vi "HapticSTM3.vi"() -> ()   [LabVIEW 2017]
uses:
  <vilib>/Analysis/baseanly.llb/Mean (DBL).vi
  <userlib>/PositionDLL/PositionDLL.lvlib
  <userlib>/Nanonis Prog Interface V5/Nanonis Prog Interface.lvlib
  <vilib>/Analysis/NI_AALBase.lvlib
panel:
  in  "mean":dbl
  in  "Averaging Done?":bool
  out "Numeric":i32
  out "PLANE HEIGHT":dbl
  out "Current":dbl
  out "Input Z":dbl
  out "Origin Y":dbl
  out "Origin X":dbl
  out "Output Z":dbl
  in  "Rough adjust":dbl
  out "Nano Z":dbl
  out "Y Out":dbl
  out "X Out":dbl
  out "Max speed":dbl
  out "Width":dbl
  out "VY":dbl
  out "VZ":dbl
  out "VX":dbl
  in  "Drag":dbl=1.0
  in  "STOP":bool
  in  "START":bool
  out "Fy":dbl
  out "Fz":dbl
  out "phi":dbl
  out "psi":dbl
  out "Fx":dbl
  out "theta":dbl
  out "x":dbl
  out "y":dbl
  out "z":dbl
  in  "Fine adjust":dbl=3.5
  out "Clicks":dbl
  out "Height":dbl
  # "Sample Window"
  # "Position"
  # "Sensitivity"
  # "Force"
  # "STM I/O"
  # "Angles"
  # "Velocity"
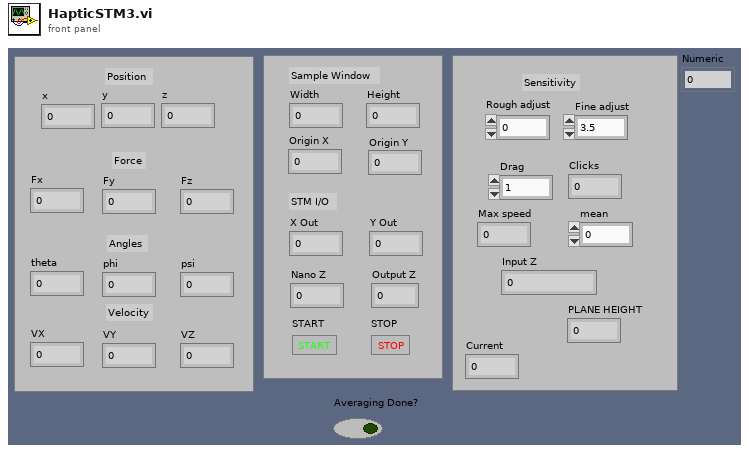
[diagram p1: front panel]
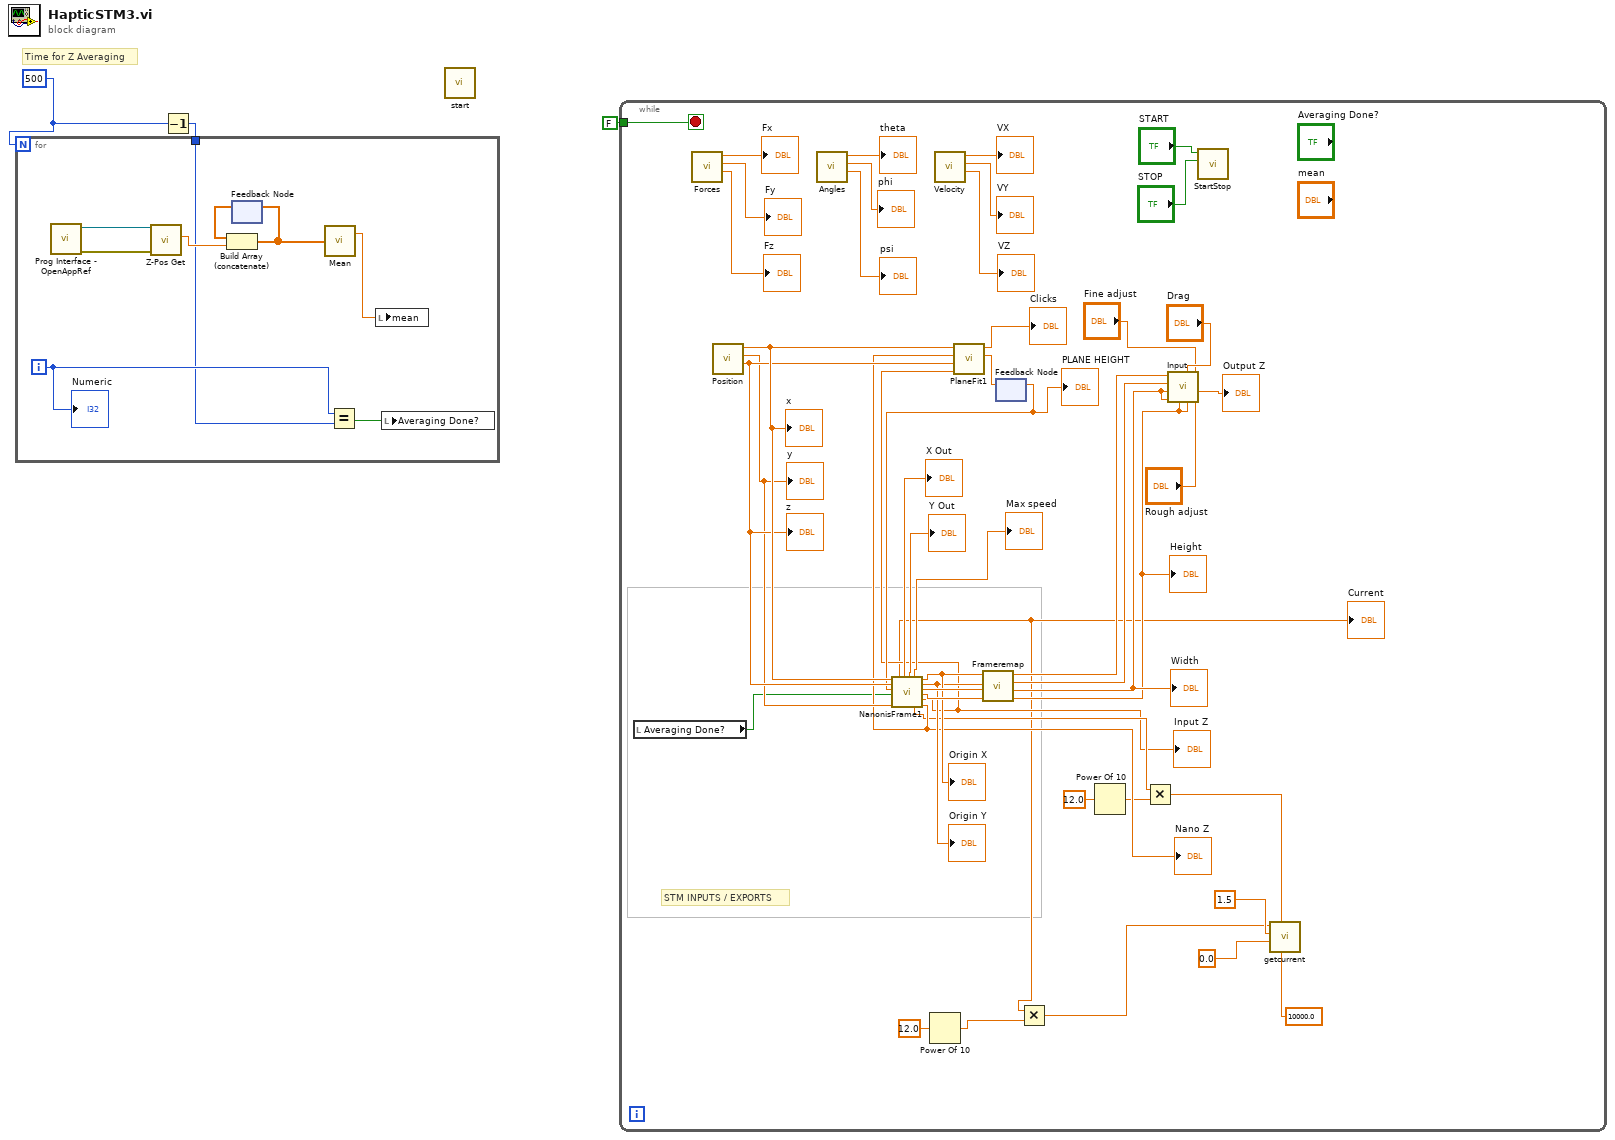
[diagram p0: block diagram]
diagram:
  w2 = 500
  # "Time for Z Averaging"
  n1 = Decrement(x=w2) -> (x-1=w1:i32)
  n2 = for {
    N: w2 -> [_]
    tunnel: w1 -> [w5]
    i -> [w7]
    n3 = call <userlib>:"Prog Interface - OpenAppRef.vi"() -> ("Error out"=w11:errorcluster, "Application reference"=w12:refnum<vi>)  [unwired: 6 in]
    n4 = call <userlib>:"Z-Pos Get.vi"("error in (no error)"=w11, "Application ref in"=w12) -> ("Z position (m)"=w9:sgl)  [unwired: 7 in, 2 out]
    n5 = feedback #1() -> (w10:sgl[])  [unwired: 1 in]
    n6 = Build Array (concatenate)(w10, w9) -> (w8:sgl[])
    n7 = feedback-in #1(w8) -> ()
    n8 = call-poly <vilib>:"Mean.vi"("X"=w8) -> ("mean"=w4:dbl)  [unwired: 1 out]
    n9 = Equal?(x=w7, y=w5) -> (x = y?=w6:bool)
    n10 = local write "mean"(w4) -> ()
    n11 = local write "Averaging Done?"(w6) -> ()
    "Numeric" <- w7
  }
  n12 = call <userlib>:"start.vi"() -> ()  [unwired: 11 in, 1 out]
  n13 = while {
    tunnel: FALSE -> [w50]
    stop <- w50 stop-if-true
    # "STM INPUTS / EXPORTS"
    n14 = local read "Averaging Done?"() -> (w22:bool)
    n15 = call <userlib>:"Forces.vi"() -> ("Fz"=→"Fz":dbl, "Fy"=→"Fy":dbl, "Fx"=→"Fx":dbl)  [unwired: 9 in]
    n16 = call <userlib>:"Position.vi"() -> ("Z"=w40:dbl, "Y"=w30:dbl, "X"=w41:dbl)  [unwired: 9 in]
    "x" <- w41
    "y" <- w30
    "z" <- w40
    n17 = call <userlib>:"Angles.vi"() -> ("psi"=→"psi":dbl, "phi"=→"phi":dbl, "theta"=→"theta":dbl)  [unwired: 9 in]
    n18 = Power Of 10(x=12.0) -> (10^x=w17:dbl)
    n19 = call <userlib>:"Velocity.vi"() -> ("VZ"=→"VZ":dbl, "VY"=→"VY":dbl, "VX"=→"VX":dbl)  [unwired: 9 in]
    n20 = feedback #2() -> (w26:dbl)  [unwired: 1 in]
    "PLANE HEIGHT" <- w26
    n21 = call <userlib>:"NanonisFrame1.vi"("x"=w41, "z"=w40, "Plane Height"=w26, "Avg Done?"=w22, "Y"=w30) -> ("Current"=w14:dbl, "X Out"=→"X Out":dbl, "Z Out"=→"Y Out":dbl, "Speed"=→"Max speed":dbl, "Setpoint Current"=w19:dbl, "FO X"=w32:dbl, "FO Z"=w31:dbl, "FW"=w36:dbl, "FH"=w35:dbl, "TIP Z"=w15:dbl, "Z position (nm)"=w29:sgl)  [unwired: 4 in]
    "Nano Z" <- w29
    "Origin X" <- w32
    "Origin Y" <- w31
    "Input Z" <- w15
    "Current" <- w14
    n22 = call <userlib>:"PlaneFit1.vi"("Y PEN"=w15, "Z"=w40, "Nano Z"=w29, "X"=w41) -> ("Output"=w27:dbl, "Clicks"=→"Clicks":dbl)  [unwired: 6 in]
    n23 = call <userlib>:"Frameremap.vi"("FH"=w35, "FW"=w36, "FO Z"=w31, "FO X"=w32) -> ("FH"=w42:dbl, "FW"=w43:dbl, "Z Origin"=w52:dbl, "X Origin"=w53:dbl)  [unwired: 4 in]
    "Height" <- w42
    "Width" <- w43
    n24 = feedback-in #2(w27) -> ()
    n25 = Multiply(x=w14, y=w17) -> (x*y=w13:dbl)
    n26 = Power Of 10(x=12.0) -> (10^x=w21:dbl)
    n27 = Multiply(x=w19, y=w21) -> (x*y=w18:dbl)
    n28 = call <userlib>:"Input.vi"("Current * 10^input"="Rough adjust", "Sensitivity"="Fine adjust", "Scopez"=w42, "Drag"="Drag", "FH"=w42, "FW"=w43, "Scopex"=w43, "Z origin"=w52, "X origin"=w53) -> ("Scaled Current"=→"Output Z":dbl)  [unwired: 2 in]
    n29 = call <userlib>:"StartStop.vi"("STOP"="STOP", "START"="START") -> ()  [unwired: 10 in]
    n30 = call <userlib>:"getcurrent.vi"("maxcurrentin"=10000.0, "setpoint"=w18, "minforcey"=0.0, "maxforcey"=1.5, "currentin"=w13) -> ()  [unwired: 7 in]
  }
